vi "MBUS_GetExceptionCode.vi"(11 "inputData":u8[](array[numeric])) -> (2 "ModbusExceptionCode":u8, 3 "ModbusException":bool=TRUE)   [LabVIEW 2012, in "MBUS_Modbus.lvlib"]
uses:
  MBUS_Modbus.lvlib
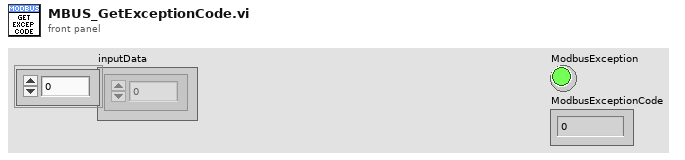
[diagram p1: front panel]
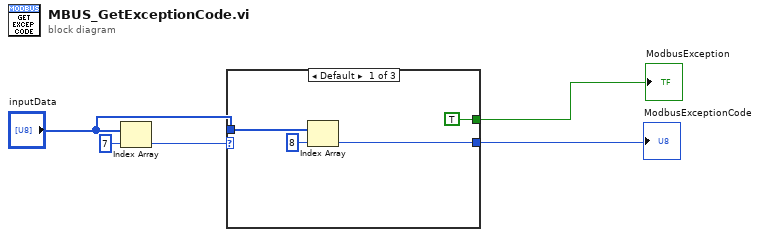
[diagram p0: block diagram]
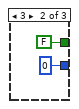
[diagram p2: hidden frame]
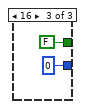
[diagram p3: hidden frame]
diagram:
  n1 = Index Array(array="inputData", index=7) -> (element=w4:u8)
  n2 = case shown="Default" w4 {
    tunnel: "inputData" -> [w9 _ _]
    tunnel: [w7 u8 0 ("Numeric Control") u8 0 ("Numeric Control")] -> w1
    tunnel: [TRUE ("ModbusException") FALSE ("ModbusException") FALSE ("ModbusException")] -> w2
    frame Default {
      n3 = Index Array(array=w9, index=8) -> (element=w7:u8)
    }
    frame 3 {
    }
    frame 16 {
    }
  }
  "ModbusException" <- w2
  "ModbusExceptionCode" <- w1
